vi "WiFi Library Example.vi"() -> ()   [LabVIEW 2012]
doc: "This VI demonstrates the use of \"WiFi Library for LabVIEW\"."
panel:
  in  "XML Input":string
  in  "XML Write":bool
  in  "Show Profiles":bool
  in  "Auth Encr":bool
  in  "Connect":bool
  out "Log Window":string
  in  "XML Path":path
  in  "Password":string
  in  "Show Networks":bool
  in  "Export Profile":bool
  in  "Delete Profile":bool
  in  "Add Profile":bool
  in  "Disconnect":bool
  in  "Network":i32(ring) items=["HackersNet"]
  in  "stop":bool
  # "Overview:\nThis VI demonstrates the use of \"WiFi Library for LabVIEW\".\nRequirements:\n1. WiFi Library for LabVIEW\n2 LabVIEW 2012 (or compatible)\n3. Windows 7 (or compatible)\n4. Computer with wireless adapter \nInstructions:\n1. Add Profile - Adds a WLAN profile to the specified interface on the computer.\n2. Connect - Connects to a wireless network by using the specified parameter.\n3. Custom XML Write - Writes XML files without the <LVData> header.\n4. Delete Profile - Removes a WLAN profile from one or multiple interfaces.\n5. Disconnect - Disconnects the specified interface from a wireless network.\n6. Export Profile - Saves WLAN profiles as XML files to the specified location.\n7. Get Authentication Encryption - Returns the authentication and encryption type.\n8. Show Networks - Displays a list of wireless networks that are visible on the computer.\n9. Show Profiles - Displays a list of wireless profiles that are configured on the computer.\n10. Enjoy WiFi!"
  # "Control Buttons"
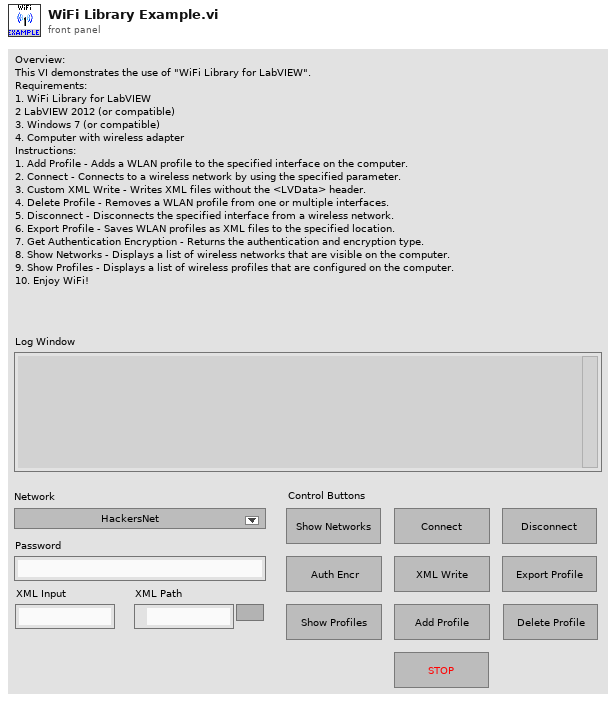
[diagram p1: front panel]
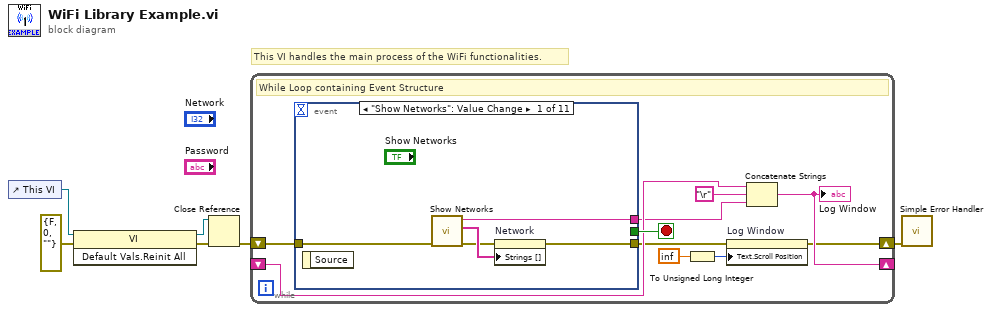
[diagram p0: block diagram]
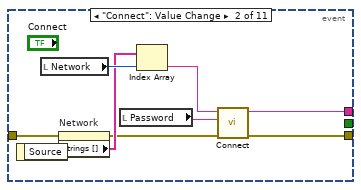
[diagram p2: hidden frame]
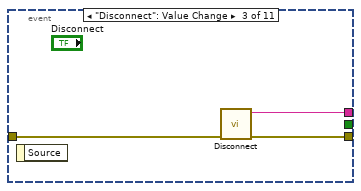
[diagram p3: hidden frame]
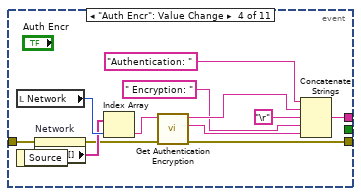
[diagram p4: hidden frame]
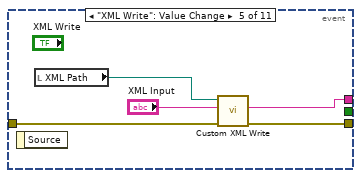
[diagram p5: hidden frame]
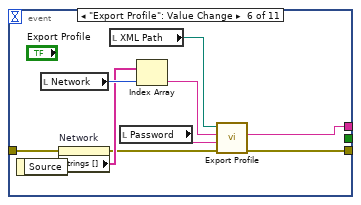
[diagram p6: hidden frame]
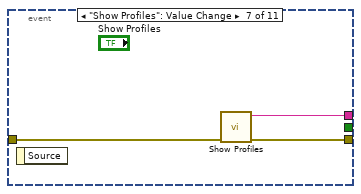
[diagram p7: hidden frame]
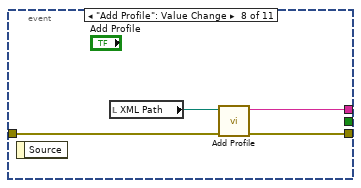
[diagram p8: hidden frame]
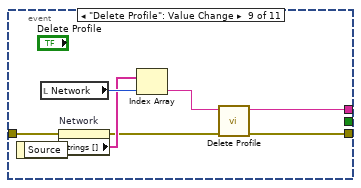
[diagram p9: hidden frame]
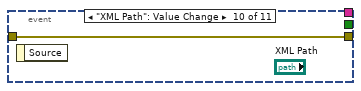
[diagram p10: hidden frame]
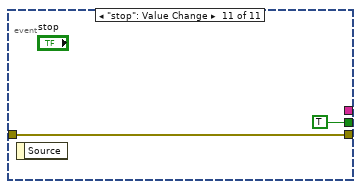
[diagram p11: hidden frame]
diagram:
  # "This VI handles the main process of the WiFi functionalities."
  n1 = control-ref of="This VI"() -> (w6:refnum<vi>)
  n2 = invoke class="VI" method="Default Vals.Reinit All"(reference=w6, error in=errorcluster {"status"=FALSE, "code"=0, "source"=""} ("error out")) -> (reference out=w4:refnum<vi>, error out=w5:errorcluster)  [unwired: 1 in, 1 out]
  n3 = Close Reference(reference=w4, error in (no error)=w5) -> (error out=w2:errorcluster)
  n4 = while {
    shift-right: [w9] -> w1
    shift-left: w2 -> [w15]
    shift-right: [w14] -> _
    shift-left: _ -> [w13]
    stop <- w16 stop-if-true
    # "While Loop containing Event Structure"
    n5 = event shown="[0] \"Show Networks\": Value Change" {
      selector: _ -> [_ _ _ _ _ _ _ _ _ _ _]
      dyn-events: _ -> [_ _ _ _ _ _ _ _ _ _ _]
      timeout: _ -> [_ _ _ _ _ _ _ _ _ _ _]
      tunnel: [_ _ _ _ _ _ _ _ _ _ TRUE] -> w16
      tunnel: w15 -> [w21 w22 w32 w42 w47 w53 w60 w64 w69 w73 w74]
      tunnel: [w17 w24 w31 w39 w45 w51 w61 w63 w67 w73 w74] -> w10
      tunnel: [w20 w23 w30 w38 w46 w50 w59 w62 w66 _ _] -> w11
      event "Show Networks": Value Change {
        n6 = event-data() -> ()  [unwired: 1 in, 1 out]
        n7 = call "Show Networks.vi"("error in (no error)"=w21) -> ("error out"=w18:errorcluster, "SSID"=w19:string[], "Feedback"=w20:string)  [unwired: 8 in]
        n8 = property on="Network" class="Ring (strict)"(error in=w18, "Strings []"=w19) -> (error out=w17:errorcluster)  [unwired: 1 in, 1 out]
      }
      event "Connect": Value Change {
        n9 = event-data() -> ()  [unwired: 1 in, 1 out]
        n10 = local read "Network"() -> (w29:i32)
        n11 = property on="Network" class="Ring (strict)"(error in=w22) -> (error out=w25:errorcluster, "Strings []"=w28:string[])  [unwired: 1 in, 1 out]
        n12 = local read "Password"() -> (w26:string)
        n13 = Index Array(array=w28, index=w29) -> (element=w27:string)
        n14 = call "Connect.vi"("error in (no error)"=w25, "Password"=w26, "SSID"=w27) -> ("error out"=w24:errorcluster, "Feedback"=w23:string)  [unwired: 7 in]
      }
      event "Disconnect": Value Change {
        n15 = event-data() -> ()  [unwired: 1 in, 1 out]
        n16 = call "Disconnect.vi"("error in (no error)"=w32) -> ("error out"=w31:errorcluster, "Feedback"=w30:string)  [unwired: 9 in]
      }
      event "Auth Encr": Value Change {
        n17 = local read "Network"() -> (w44:i32)
        n18 = event-data() -> ()  [unwired: 1 in, 1 out]
        n19 = property on="Network" class="Ring (strict)"(error in=w42) -> (error out=w41:errorcluster, "Strings []"=w43:string[])  [unwired: 1 in, 1 out]
        n20 = Index Array(array=w43, index=w44) -> (element=w40:string)
        n21 = call "Get Authentication Encryption.vi"("error in (no error)"=w41, "SSID"=w40) -> ("error out"=w39:errorcluster, "Encryption"=w33:string, "Authentication"=w36:string)  [unwired: 7 in]
        n22 = Concatenate Strings("Authentication: " ("string"), w36, "\r", " Encryption: " ("string"), w33) -> (w38:string)
      }
      event "XML Write": Value Change {
        n23 = event-data() -> ()  [unwired: 1 in, 1 out]
        n24 = local read "XML Path"() -> (w49:path)
        n25 = call "Custom XML Write.vi"("error in (no error)"=w47, "XML Input"="XML Input", "XML File Path"=w49) -> ("error out"=w45:errorcluster, "XML String"=w46:string)  [unwired: 6 in, 1 out]
      }
      event "Export Profile": Value Change {
        n26 = event-data() -> ()  [unwired: 1 in, 1 out]
        n27 = local read "Network"() -> (w57:i32)
        n28 = property on="Network" class="Ring (strict)"(error in=w53) -> (error out=w52:errorcluster, "Strings []"=w56:string[])  [unwired: 1 in, 1 out]
        n29 = local read "XML Path"() -> (w58:path)
        n30 = local read "Password"() -> (w54:string)
        n31 = Index Array(array=w56, index=w57) -> (element=w55:string)
        n32 = call "Export Profile.vi"("error in (no error)"=w52, "Password"=w54, "SSID"=w55, "XML path in"=w58) -> ("error out"=w51:errorcluster, "Feedback"=w50:string)  [unwired: 5 in, 1 out]
      }
      event "Show Profiles": Value Change {
        n33 = event-data() -> ()  [unwired: 1 in, 1 out]
        n34 = call "Show Profiles.vi"("error in (no error)"=w60) -> ("error out"=w61:errorcluster, "Feedback"=w59:string)  [unwired: 9 in]
      }
      event "Add Profile": Value Change {
        n35 = event-data() -> ()  [unwired: 1 in, 1 out]
        n36 = local read "XML Path"() -> (w65:path)
        n37 = call "Add Profile.vi"("error in (no error)"=w64, "Path"=w65) -> ("error out"=w63:errorcluster, "Feedback"=w62:string)  [unwired: 8 in]
      }
      event "Delete Profile": Value Change {
        n38 = event-data() -> ()  [unwired: 1 in, 1 out]
        n39 = local read "Network"() -> (w72:i32)
        n40 = property on="Network" class="Ring (strict)"(error in=w69) -> (error out=w68:errorcluster, "Strings []"=w71:string[])  [unwired: 1 in, 1 out]
        n41 = Index Array(array=w71, index=w72) -> (element=w70:string)
        n42 = call "Delete Profile.vi"("error in (no error)"=w68, "SSID"=w70) -> ("error out"=w67:errorcluster, "Feedback"=w66:string)  [unwired: 8 in]
      }
      event "XML Path": Value Change {
        n43 = event-data() -> ()  [unwired: 1 in, 1 out]
      }
      event "stop": Value Change {
        n44 = event-data() -> ()  [unwired: 1 in, 1 out]
      }
    }
    n45 = To Unsigned Long Integer(number=inf) -> (unsigned 32bit integer=w7:u32)
    n46 = property on="Log Window" class="Str"(error in=w10, "Text.Scroll Position"=w7) -> (error out=w9:errorcluster)  [unwired: 1 in, 1 out]
    n47 = Concatenate Strings(w13, "\r", w11) -> (w14:string)
    "Log Window" <- w14
  }
  n48 = call <vilib>:"Simple Error Handler.vi"("error in (no error)"=w1) -> ()  [unwired: 4 in, 5 out]
